vi "FPGA Acknowledge IRQ.vi"(8 "error in (no error)":errorcluster, 10 "IRQ":u32, 11 "FPGA Session In":refnum<class "FPGA Interface Base.lvclass">) -> (0 "error out":errorcluster, 3 "FPGA Session Out":refnum<class "FPGA Interface Base.lvclass">)   [LabVIEW 2010, in "FPGA Interface Base.lvclass"]
uses:
  <userlib>/_FPGA Interface Advanced Tools/FPGA Interface Base/FPGA Interface Base.lvclass
  <userlib>/_FPGA Interface Advanced Tools/FPGA Interface Base/Accessors/FPGA Read Session.vi
  <vilib>/Utility/error.llb/Error Cluster From Error Code.vi
  <userlib>/_FPGA Interface Advanced Tools/FPGA Interface Wrapper/FPGA Interface Wrapper.lvlib
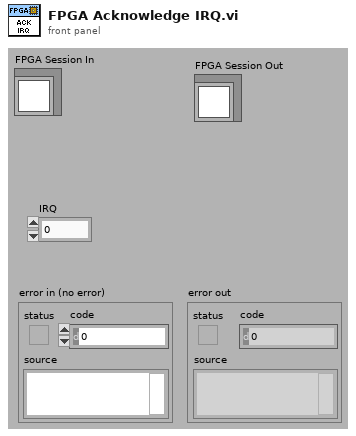
[diagram p1: front panel]
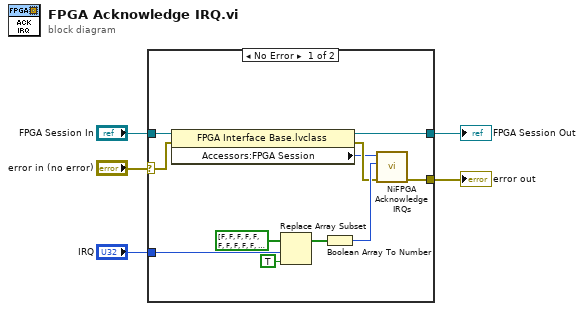
[diagram p0: block diagram]
diagram:
  n1 = case shown="No Error" "error in (no error)" {
    selector: "error in (no error)" -> [w10 w18]
    tunnel: [w6 w18] -> w2
    tunnel: [w7 w17] -> w4
    tunnel: "FPGA Session In" -> [w11 w17]
    tunnel: "IRQ" -> [w14 _]
    frame No Error {
      n2 = property class="FPGA Interface Base.lvclass"(reference=w11, error in=w10) -> (reference out=w7:refnum<class "FPGA Interface Base.lvclass">, error out=w9:errorcluster, "Accessors:FPGA Session"=w8:u32)
      n3 = Replace Array Subset(array=bool[] [FALSE, FALSE, FALSE, FALSE, FALSE, FALSE, FALSE, FALSE, FALSE, FALSE, FALSE, FALSE, FALSE, FALSE, FALSE, FALSE, FALSE, FALSE, FALSE, FALSE, FALSE, FALSE, FALSE, FALSE, FALSE, FALSE, FALSE, FALSE, FALSE, FALSE, FALSE, FALSE], new element=TRUE ("new element/subarray"), index=w14) -> (w16:bool[])
      n4 = Boolean Array To Number(Boolean array=w16) -> (number=w13:u32)
      n5 = call <userlib>:"NiFPGA Acknowledge IRQs.vi"("error in (no error)"=w9, "IRQs"=w13, "Session In"=w8) -> ("error out"=w6:errorcluster)  [unwired: 7 in, 1 out]
    }
    frame Error {
    }
  }
  "error out" <- w2
  "FPGA Session Out" <- w4
